vi "Stay or Go.vi"(8 "error in (no error)":errorcluster) -> ()   [LabVIEW 2009]
panel:
  # "VI determines if application is executable or not. If it is executable it exits LabView when called so the panel\nis not laeft on the computer screen."
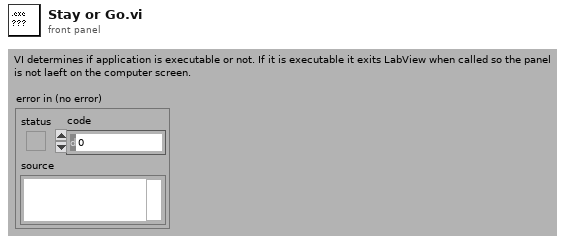
[diagram p1: front panel]
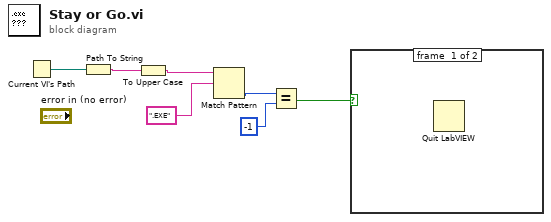
[diagram p0: block diagram]
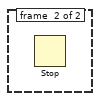
[diagram p2: hidden frame]
diagram:
  n1 = Current VI's Path() -> (path=w7:path)
  n2 = Path To String(path=w7) -> (string=w6:string)
  n3 = To Upper Case(1:w6) -> (0:w5:string)
  n4 = Match Pattern(string=w5, regular expression=".EXE") -> (offset past match=w3:i32)  [unwired: 4 out]
  n5 = Equal?(x=w3, y=-1) -> (x = y?=w1:bool)
  n6 = case shown="True" w1 {
    frame #0 {
      n7 = Quit LabVIEW() -> ()  [unwired: 1 out]
    }
    frame #1 {
      n8 = Stop() -> ()  [unwired: 1 out]
    }
  }
